vi "ShowFlyout.vi"(7 "MainUI":refnum<queue>, 8 "error in (no error)":errorcluster, 9 "Subpanel":refnum<vi>, 10 "Timeout":dbl, 11 "Message":string) -> (0 "error out":errorcluster)   [LabVIEW 2019, in "Flyout.lvlib"]
uses:
  Flyout.lvlib
  MainController/Cluster - MainControllerMessage.ctl
  MainController/Enum - MainState.ctl
  Flyout.vi
  support/User Interface/UserInterface.lvlib
  MainController/MainController.lvlib
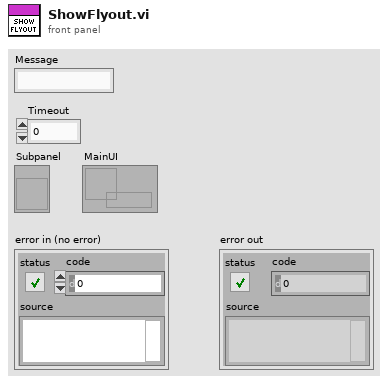
[diagram p1: front panel]
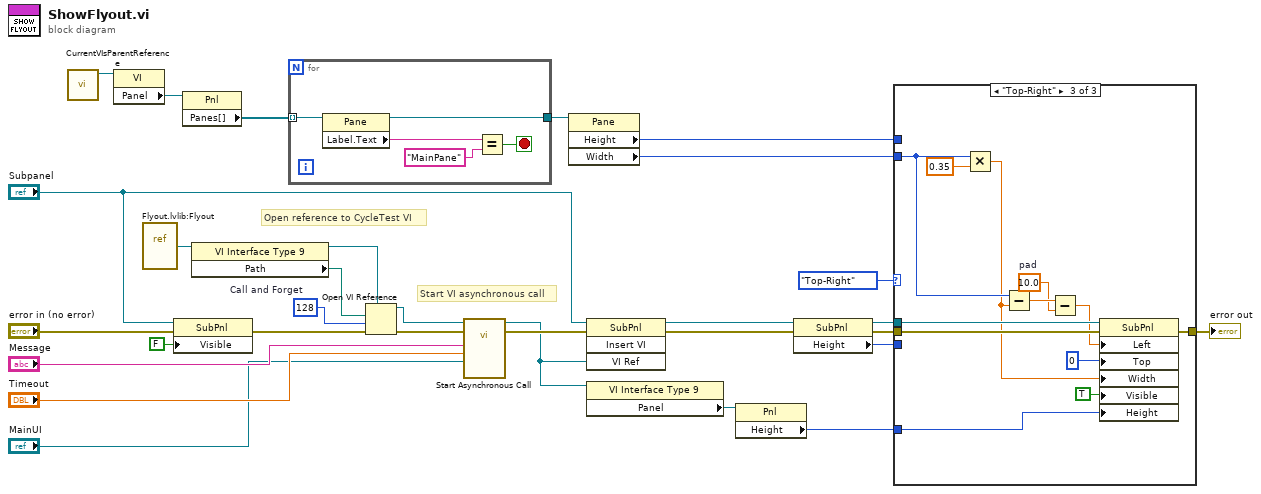
[diagram p0: block diagram]
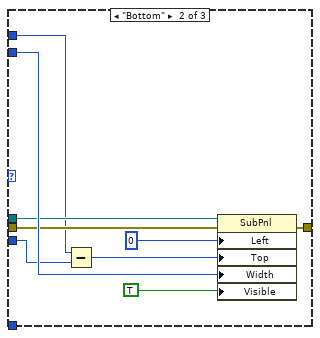
[diagram p3: hidden frame]
diagram:
  w26 = 128  # Call and Forget
  # "Start VI asynchronous call"
  # "Open reference to CycleTest VI"
  n1 = call "CurrentVIsParentReference.vi"() -> ("ParentVIReference"=w1:refnum<vi>)  [unwired: 11 in]
  n2 = property class="VI"(reference=w1) -> ("Panel"=w16:refnum<vi>)  [unwired: 1 in, 2 out]
  n3 = vi-ref "Flyout.lvlib:Flyout.vi"() -> (w27:refnum<vi>)
  n4 = property class="SubPnl"(reference="Subpanel", error in="error in (no error)", "Visible"=FALSE) -> (error out=w20:errorcluster)  [unwired: 1 out]
  n5 = property class="Pnl"(reference=w16) -> ("Panes[]"=w15:refnum<vi>[])  [unwired: 1 in, 2 out]
  n6 = property class="VI Interface Type 9"(reference=w27) -> (reference out=w25:refnum<vi>, "Path"=w30:path)  [unwired: 1 in, 1 out]
  n7 = for {
    tunnel: w15 -> [w35] mode=indexing
    tunnel: [w31] -> w14
    stop <- w32 stop-if-true
    n8 = property class="Pane"(reference=w35) -> (reference out=w31:refnum<vi>, "Label.Text"=w34:string)  [unwired: 1 in, 1 out]
    n9 = Equal?(x=w34, y="MainPane") -> (x = y?=w32:bool)
  }
  n10 = Open VI Reference(type specifier VI Refnum (for type only)=w25, vi path=w30, options=w26, error in (no error)=w20) -> (vi reference=w29:refnum<vi>, error out=w28:errorcluster)  [unwired: 2 in]
  n11 = call-by-ref "Start Asynchronous Call"(reference=w29, error in=w28, "Message Queue"="MainUI", "Timeout"="Timeout", "Message"="Message") -> (reference out=w4:refnum<vi>, error out=w21:errorcluster)  [unwired: 8 in, 1 out]
  n12 = property class="Pane"(reference=w14) -> ("Height"=w7:u32, "Width"=w13:u32)  [unwired: 1 in, 2 out]
  n13 = invoke class="SubPnl" method="Insert VI"(reference="Subpanel", error in=w21, "VI Ref"=w4) -> (reference out=w11:refnum<vi>, error out=w12:errorcluster)  [unwired: 1 in, 2 out]
  n14 = property class="VI Interface Type 9"(reference=w4) -> ("Panel"=w3:refnum<vi>)  [unwired: 1 in, 2 out]
  n15 = property class="Pnl"(reference=w3) -> ("Height"=w2:u32)  [unwired: 1 in, 2 out]
  n16 = property class="SubPnl"(reference=w11, error in=w12) -> (reference out=w9:refnum<vi>, error out=w10:errorcluster, "Height"=w8:u32)
  n17 = case shown="\"Top-Right\"" enum16{"Bottom", "Top-Right"}."Top-Right" {
    tunnel: [w36 w45 w57] -> w17
    tunnel: w13 -> [_ w43 w51]
    tunnel: w10 -> [w36 w41 w55]
    tunnel: w9 -> [_ w40 w54]
    tunnel: w8 -> [_ w39 _]
    tunnel: w7 -> [_ w38 _]
    tunnel: w2 -> [_ _ w49]
    frame Default {
    }
    frame "Bottom" {
      n18 = Subtract(x=w38, y=w39) -> (x-y=w37:u32)
      n19 = property class="SubPnl"(reference=w40, error in=w41, "Left"=0 ("Position:Left"), "Top"=w37, "Width"=w43, "Visible"=TRUE) -> (error out=w45:errorcluster)  [unwired: 1 out]
    }
    frame "Top-Right" {
      w47 = 10.0  # pad
      n20 = Multiply(x=w51, y=0.35) -> (x*y=w50:dbl)
      n21 = Subtract(x=w51, y=w50) -> (x-y=w48:dbl)
      n22 = Subtract(x=w48, y=w47) -> (x-y=w46:dbl)
      n23 = property class="SubPnl"(reference=w54, error in=w55, "Left"=w46, "Top"=0 ("Position:Left"), "Width"=w50, "Visible"=TRUE, "Height"=w49) -> (error out=w57:errorcluster)  [unwired: 1 out]
    }
  }
  "error out" <- w17
